vi "init_DAC_piezo_ai_chans.vi"(10 "Sample Rate":dbl) -> (0 "error out":errorcluster, 2 "Number Chans":dbl, 3 "Refnum out":refnum<k21>)   [LabVIEW 2015]
uses:
  <vilib>/DAQmx/create/channels.llb/DAQmx Create Channel (AI-Voltage-Basic).vi
  <vilib>/DAQmx/configure/timing.llb/DAQmx Timing (Sample Clock).vi
  <resource>/objmgr/daqmx.rc
panel:
  out "Actual Sample Rate":dbl=1000.0 format="%0.2f"
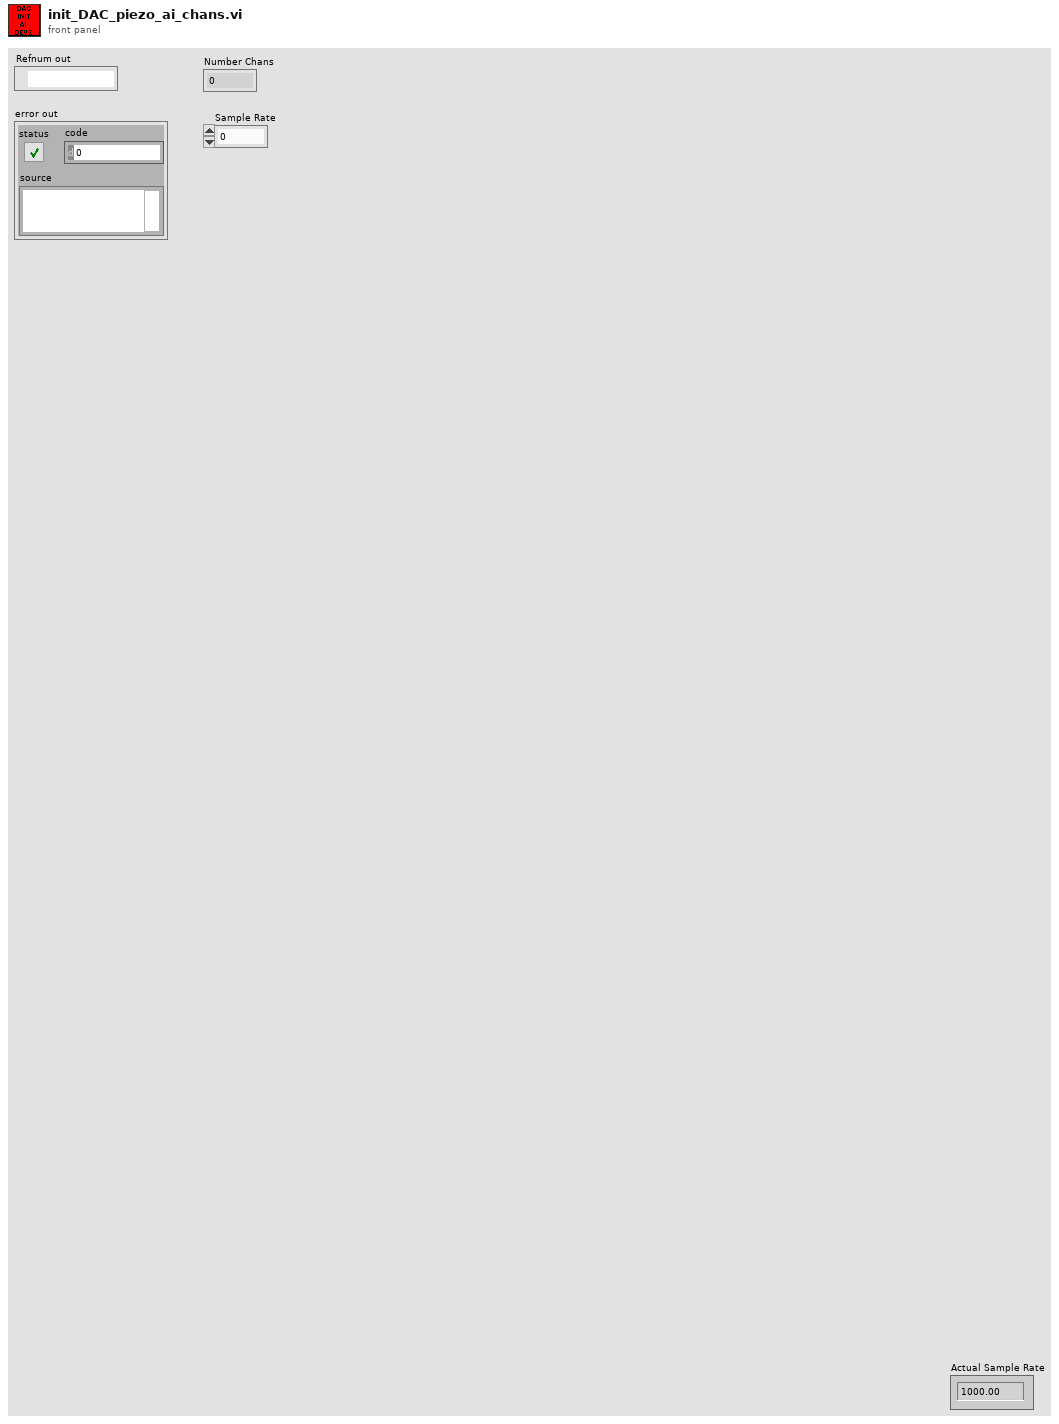
[diagram p1: front panel]
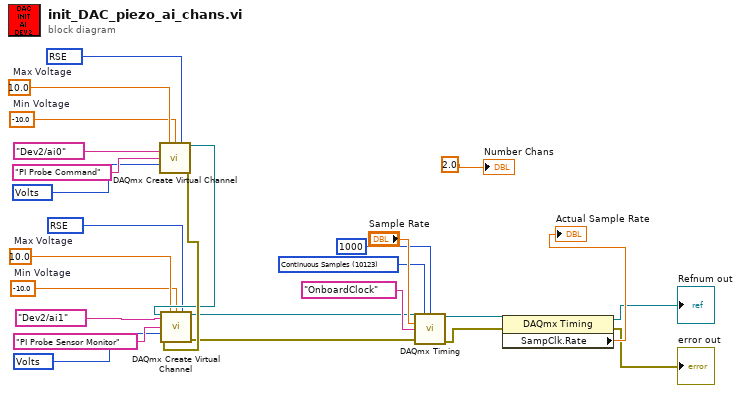
[diagram p0: block diagram]
diagram:
  w2 = 10123 items=["Finite Samples"=10178, "Continuous Samples"=10123] ("sample mode")
  w21 = 10348 items=["Volts"=10348, "From Custom Scale"=10065] ("units")
  w20 = 10083 items=["default"=-1, "RSE"=10083, "NRSE"=10078, "Differential"=10106, "Pseudodifferential"=12529] ("input terminal configuration")
  w18 = -10.0  # Min Voltage
  w19 = 10.0  # Max Voltage
  w16 = 10348 items=["Volts"=10348, "From Custom Scale"=10065] ("units")
  w15 = 10083 items=["default"=-1, "RSE"=10083, "NRSE"=10078, "Differential"=10106, "Pseudodifferential"=12529] ("input terminal configuration")
  w13 = -10.0  # Min Voltage
  w14 = 10.0  # Max Voltage
  n1 = call-poly <vilib>:"DAQmx Create Virtual Channel.vi"("maximum value"=w14, "minimum value"=w13, "input terminal configuration"=w15, "physical channels"=tag "Dev2/ai0" ("DAQmx Physical Channel"), "name to assign"="PI Probe Command", "units"=w16) -> ("task out"=w23:refnum<k21>, "error out"=w24:errorcluster)  [unwired: 8 in]
  n2 = call-poly <vilib>:"DAQmx Create Virtual Channel.vi"("task in"=w23, "maximum value"=w19, "minimum value"=w18, "input terminal configuration"=w20, "physical channels"=tag "Dev2/ai1" ("DAQmx Physical Channel"), "name to assign"="PI Probe Sensor Monitor", "units"=w21, "error in"=w24) -> ("task out"=w4:refnum<k21>, "error out"=w3:errorcluster)  [unwired: 6 in]
  n3 = call-poly <vilib>:"DAQmx Timing.vi"("task/channels in"=w4, "sample mode"=w2, "samples per channel"=1000, "rate"="Sample Rate", "source"=tag "OnboardClock" ("Sample Clock Source"), "error in"=w3) -> ("task out"=w11:refnum<k21>, "error out"=w10:errorcluster)  [unwired: 8 in]
  n4 = property class="DAQmx Timing"(reference=w11, error in=w10) -> (reference out=→"Refnum out":refnum<k21>, error out=→"error out":errorcluster, "SampClk.Rate"=→"Actual Sample Rate":dbl)
  "Number Chans" <- 2.0 ("Number Chans")
